vi "Salinity Relations.vi"(3 "Adde Vapor":dbl[unit], 4 "S2 / Salinity of Output Exposed Saline Water":dbl=0.004, 5 "S1 / Salinity of Input Exposed Saline Water":dbl=0.0035) -> (0 "S1 is greater Than S2\nThat is Wrong":bool, 1 "Output Exposed Saline Water":dbl[unit], 2 "Input Exposed Saline Water":dbl[unit])   [LabVIEW 2018]
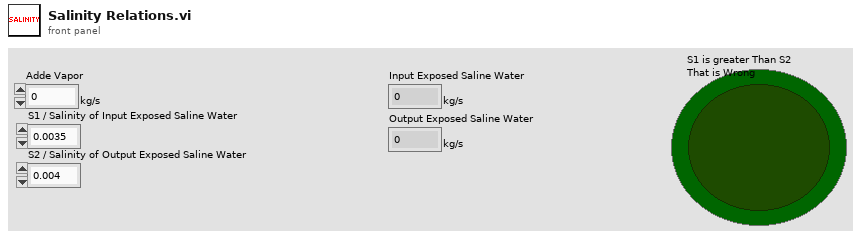
[diagram p1: front panel]
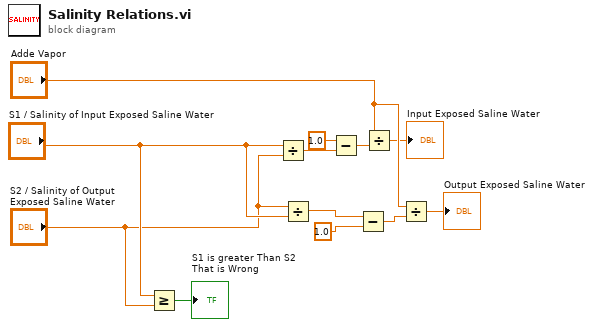
[diagram p0: block diagram]
diagram:
  n1 = Greater Or Equal?(x="S1 / Salinity of Input Exposed Saline Water", y="S2 / Salinity of Output Exposed Saline Water") -> (x >= y?=→"S1 is greater Than S2\nThat is Wrong":bool)
  n2 = Divide(x="S1 / Salinity of Input Exposed Saline Water", y="S2 / Salinity of Output Exposed Saline Water") -> (x/y=w9:dbl)
  n3 = Divide(x="S2 / Salinity of Output Exposed Saline Water", y="S1 / Salinity of Input Exposed Saline Water") -> (x/y=w8:dbl)
  n4 = Subtract(x=1.0, y=w9) -> (x-y=w11:dbl)
  n5 = Subtract(x=w8, y=1.0) -> (x-y=w7:dbl)
  n6 = Divide(x="Adde Vapor", y=w11) -> (x/y=→"Input Exposed Saline Water":dbl[unit])
  n7 = Divide(x="Adde Vapor", y=w7) -> (x/y=→"Output Exposed Saline Water":dbl[unit])
